vi "Update UI per Reference.vi"(8 "error in (no error)":errorcluster, 11 "Analyze Results Energy in":refnum<class "Analyze Results Energy.lvclass">) -> (0 "error out":errorcluster, 3 "Analyze Results Energy out":refnum<class "Analyze Results Energy.lvclass">)   [LabVIEW 2020, in "Analyze Results Energy.lvclass"]
uses:
  Analyze Results Energy.lvclass
  Analyze Results Energy.lvclass/Analyze Results Energy.ctl
  Results Total Counts/Analyze Results Total Counts.lvclass
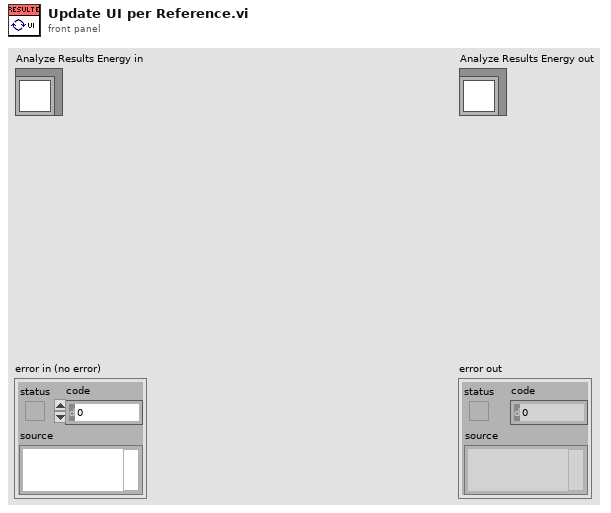
[diagram p1: front panel]
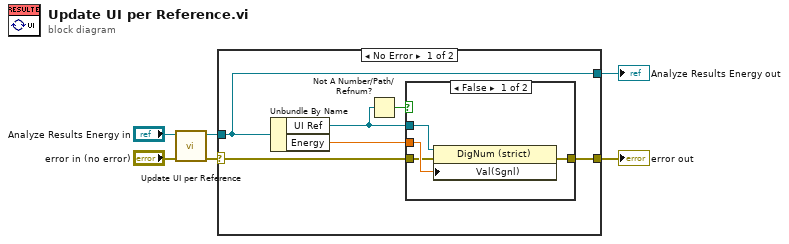
[diagram p0: block diagram]
diagram:
  n1 = call-parent "Update UI per Reference.vi"("error in (no error)"="error in (no error)", "Analyze Results Total Counts in"="Analyze Results Energy in") -> ("error out"=w2:errorcluster, "Analyze Results Total Counts out"=w4:refnum<class "Analyze Results Energy.lvclass">)  [unwired: 8 in]
  n2 = case shown="No Error" w2 {
    selector: w2 -> [w8 w19]
    tunnel: w4 -> [w7 w18]
    tunnel: [w9 w19] -> w3
    tunnel: [w7 w18] -> w1
    frame No Error {
      n3 = Unbundle By Name(w7) -> ("UI Ref"=w12:refnum<vi>, "Energy"=w11:dbl[unit])
      n4 = Not A Number/Path/Refnum?(number/path/refnum=w12) -> (NaN/Path/Refnum?=w10:bool)
      n5 = case shown="False" w10 {
        tunnel: w12 -> [w16 _]
        tunnel: w11 -> [w15 _]
        tunnel: w8 -> [w14 w17]
        tunnel: [w13 w17] -> w9
        frame False {
          n6 = property class="DigNum (strict)"(reference=w16, error in=w14, "Val(Sgnl)"=w15) -> (error out=w13:errorcluster)  [unwired: 1 out]
        }
        frame True {
        }
      }
    }
    frame Error {
    }
  }
  "error out" <- w3
  "Analyze Results Energy out" <- w1
